vi "test.workspace_create_datasource_and_connection_in_expected_workspace.vi"   [LabVIEW 2020]
uses:
  730c9c5b-7bb2-47cf-818b-6e2ed47344d4.vi
  Nominal Client/Nominal Client.lvclass
  <vilib>/addons/_JKI Toolkits/Caraya/classes/Test/Test.lvclass
  <vilib>/addons/_JKI Toolkits/Caraya/classes/Assert/Assert.lvclass
  <vilib>/addons/_JKI Toolkits/Caraya/classes/Assert/Assert Not Error.vi
  02679ea1-62f9-4fe0-ba26-58395852097e.vi
types:
  T1 = cluster{"ID":string, "RID":string, "Org":string, "Display Name":string, "Icon URL":string}[]
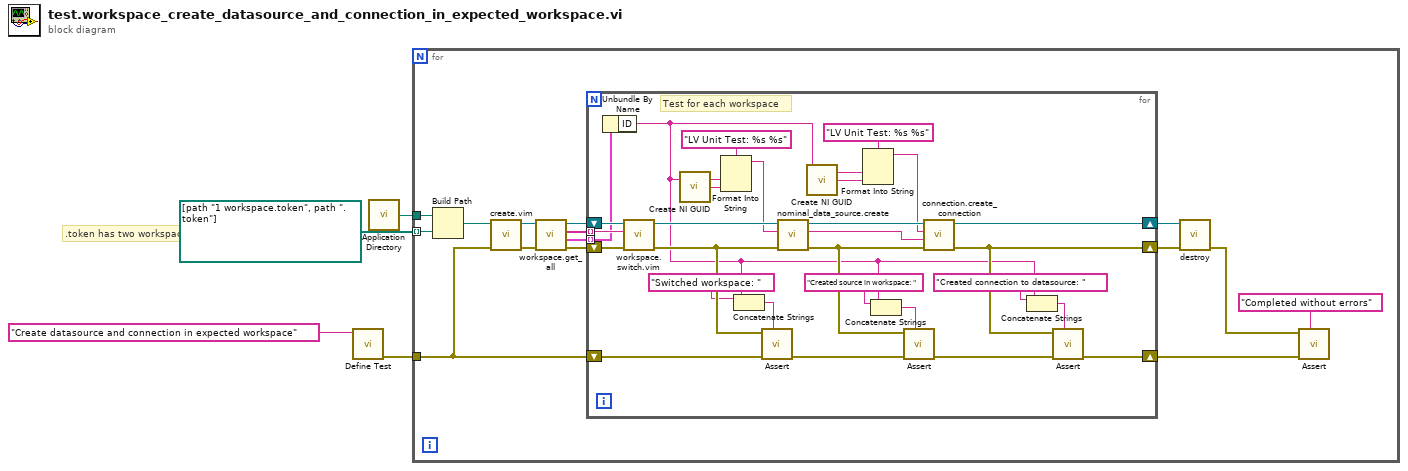
[diagram p0: block diagram]
diagram:
  # ".token has two workspaces"
  n1 = call <vilib>:"Define Test.vi"("Label (VI Title)"="Create datasource and connection in expected workspace") -> ("error out"=w3:errorcluster)  [unwired: 9 in, 1 out]
  n2 = call <vilib>:"Application Directory.vi"() -> ("Application Directory"=w2:path)
  n3 = for {
    tunnel: w3 -> [w8]
    tunnel: w2 -> [w7]
    tunnel: path[] [path "1 workspace.token", path ".token"] -> [w6] mode=indexing
    n4 = Build Path(base path=w7, name or relative path=w6) -> (appended path=w5:path)
    n5 = call "create.vim"("error in"=w8, "API Token (string or path)"=w5) -> ("error out"=w18:errorcluster, "Nominal Client"=w19:refnum<class "Nominal Client.lvclass">)  [unwired: 8 in]
    n6 = call "workspace.get_all.vi"("error in"=w18, "Nominal Client in"=w19) -> ("error out"=w15:errorcluster, "Workspace Details"=w12:T1, "Workspace RIDs"=w13:string[], "Nominal Client out"=w17:refnum<class "Nominal Client.lvclass">)  [unwired: 5 in, 1 out]
    n7 = for {
      shift-right: [w29] -> w16
      shift-left: w17 -> [w47]
      shift-right: [w28] -> w14
      shift-left: w15 -> [w45]
      tunnel: w13 -> [w46] mode=indexing
      shift-right: [w30] -> w10
      shift-left: w8 -> [w44]
      tunnel: w12 -> [w40] mode=indexing
      # "Test for each workspace"
      n8 = Unbundle By Name(w40) -> ("ID"=w20:string)
      n9 = call "workspace.switch.vim"("error in"=w45, "Workspace RID (string or path)"=w46, "Nominal Client in"=w47) -> ("error out"=w42:errorcluster, "Nominal Client out"=w43:refnum<class "Nominal Client.lvclass">)  [unwired: 7 in]
      n10 = call <vilib>:"Create NI GUID.vi"() -> ("NI GUID"=w39:string)
      n11 = Format Into String(format string="LV Unit Test: %s %s", w20, w39) -> (resulting string=w38:string)  [unwired: 2 in, 1 out]
      n12 = Concatenate Strings("Switched workspace: " ("Label"), w20) -> (w26:string)
      n13 = call-poly <vilib>:"Assert.vi"("Label"=w26, "error in (no error)"=w44, "Not Error?"=w42) -> ("error out"=w37:errorcluster)  [unwired: 7 in, 1 out]
      n14 = call "nominal_data_source.create.vi"("error in"=w42, "Name"=w38, "Nominal Client in"=w43) -> ("error out"=w21:errorcluster, "rid"=w35:string, "Nominal Client out"=w36:refnum<class "Nominal Client.lvclass">)  [unwired: 5 in, 1 out]
      n15 = call <vilib>:"Create NI GUID.vi"() -> ("NI GUID"=w34:string)
      n16 = Format Into String(format string="LV Unit Test: %s %s", w20, w34) -> (resulting string=w32:string)  [unwired: 2 in, 1 out]
      n17 = Concatenate Strings("Created source in workspace: " ("Label"), w20) -> (w24:string)
      n18 = call-poly <vilib>:"Assert.vi"("Label"=w24, "error in (no error)"=w37, "Not Error?"=w21) -> ("error out"=w31:errorcluster)  [unwired: 7 in, 1 out]
      n19 = call "connection.create_connection.vi"("error in"=w21, "nominalDataSourceRid"=w35, "name"=w32, "Nominal Client in"=w36) -> ("error out"=w28:errorcluster, "Nominal Client out"=w29:refnum<class "Nominal Client.lvclass">)  [unwired: 4 in, 2 out]
      n20 = Concatenate Strings("Created connection to datasource: " ("Label"), w20) -> (w22:string)
      n21 = call-poly <vilib>:"Assert.vi"("Label"=w22, "error in (no error)"=w31, "Not Error?"=w28) -> ("error out"=w30:errorcluster)  [unwired: 7 in, 1 out]
    }
    n22 = call "destroy.vi"("error in"=w14, "Nominal Client"=w16) -> ("error out"=w9:errorcluster)  [unwired: 9 in]
    n23 = call-poly <vilib>:"Assert.vi"("Label"="Completed without errors", "error in (no error)"=w10, "Not Error?"=w9) -> ()  [unwired: 7 in, 2 out]
  }
